vi "Write Front Panel of Function.vi"(8 "error in (no error)":errorcluster, 10 "Front Panel of Function":refnum<vi>, 11 "Function in":refnum<class "Function.lvclass">) -> (0 "error out":errorcluster, 3 "Function out":refnum<class "Function.lvclass">)   [LabVIEW 2016, in "Function Actor.lvlib" / "Function.lvclass"]
uses:
  <userlib>/Common Components/Function Actor/Function.lvclass
  <userlib>/Common Components/Function Actor/Function.lvclass/Function.ctl
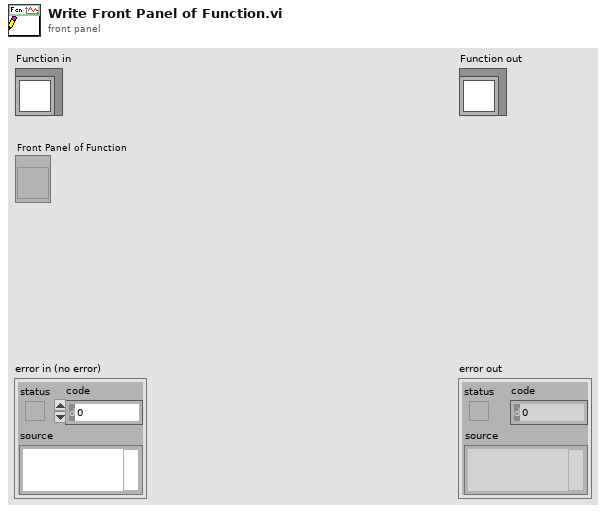
[diagram p1: front panel]
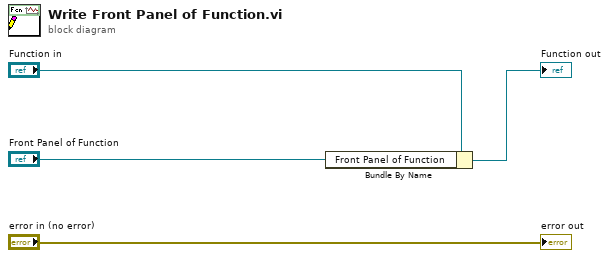
[diagram p0: block diagram]
diagram:
  n1 = Bundle By Name(cluster="Function in", "Front Panel of Function"="Front Panel of Function") -> (→"Function out":refnum<class "Function.lvclass">)
  "error out" <- "error in (no error)"
